vi "XIPIN_Utility_Vector_Logic_2_0.vi"   [LabVIEW 2017]
doc: "Performs bitwise logic operations on two n-bit inputs to produce a single n-bit output\n------------------------------------\n<b>Need License</b> : No"
uses:
  <vilib>/rvi/XilinxIP/XIPIN_XNode/niFpgaXIPIN.xnode
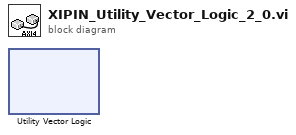
[diagram p0: block diagram]
diagram:
  n1 = xnode ("Utility Vector Logic")() -> ()
